vi "总磷氨氮MB_api.vi"(6 "Slave ID":u8=1, 7 "STEP":enum16{"open", "read", "write", "close"}(ring)=enum."read", 8 "Error in":errorcluster caption="Error in (no error)", 9 "values":u16[](array[numeric]), 10 "quantity":u16, 11 "starting address":u16 format="%04xH") -> (0 "error out":errorcluster, 2 "输出簇":T1, 3 "Registers":u16[](array[numeric]))   [LabVIEW 2016, in "氨氮.lvlib"]
uses:
  <vilib>/Plasmionique/MB Master/MB_ADU/MB_ADU.lvclass/MB_ADU.ctl
  <vilib>/Plasmionique/MB Master/MB_ADU/Read RX Data.vi
  <vilib>/Plasmionique/MB Master/MB_ADU/Read RX Timestamp.vi
  <vilib>/Plasmionique/MB Master/MB_ADU/Read Slave ID.vi
  <vilib>/Plasmionique/MB Master/MB_ADU/Read TX Data.vi
  <vilib>/Plasmionique/MB Master/MB_ADU/Read TX Timestamp.vi
  <vilib>/Plasmionique/MB Master/MB_Master_Serial/MB_Master_Serial.lvclass
  F:/Program Files/National Instruments/LabVIEW 2016/vi.lib/Plasmionique/MB Master/MB_Master/MB_Master.lvclass
  <vilib>/Plasmionique/MB Master/MB_ADU/MB_ADU.lvclass
  <vilib>/Plasmionique/MB Master/MB_Master/MB_Master.lvclass
  <vilib>/Plasmionique/MB Master/MB Master.lvlib
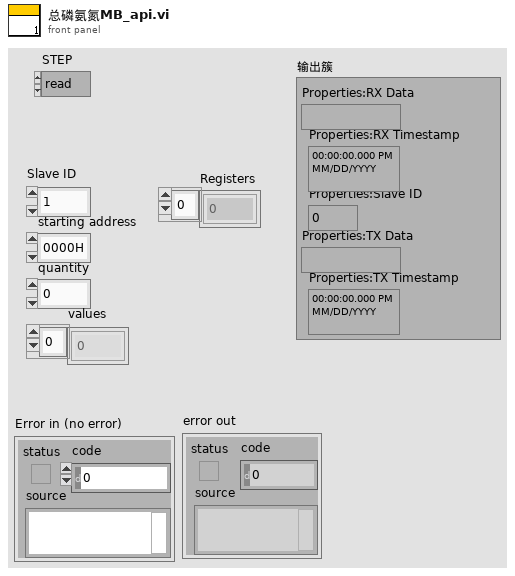
[diagram p1: front panel]
types:
  T1 = cluster{"Properties:RX Data":string, "Properties:RX Timestamp":timestamp, "Properties:Slave ID":u8, "Properties:TX Data":string, "Properties:TX Timestamp":timestamp}
  T2 = cluster{"baud rate (bps)":u32, "stop bits":u16, "parity":u16, "flow control":u16, "timeout":u32, "retries":i32}
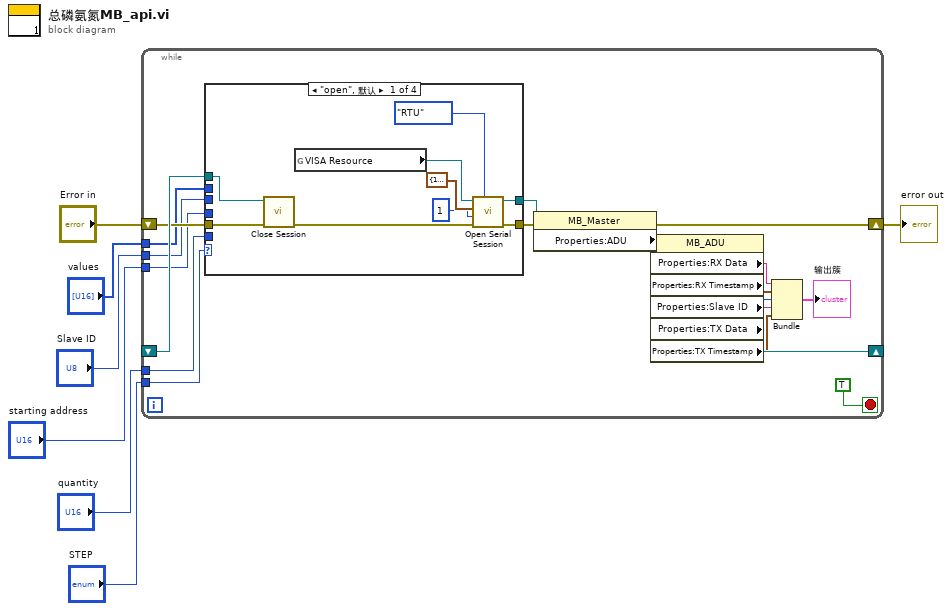
[diagram p0: block diagram]
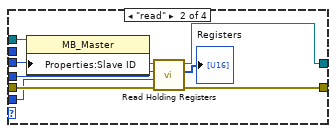
[diagram p2: hidden frame]
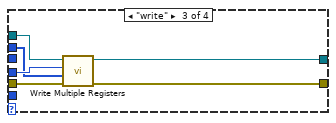
[diagram p3: hidden frame]
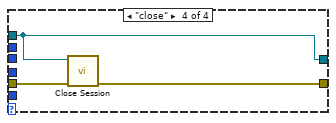
[diagram p4: hidden frame]
diagram:
  n1 = while {
    shift-right: [w19] -> _
    shift-left: _ -> [w26]
    shift-right: [w17] -> w6
    shift-left: "Error in" -> [w25]
    tunnel: "Slave ID" -> [w24]
    tunnel: "starting address" -> [w23]
    tunnel: "quantity" -> [w22]
    tunnel: "STEP" -> [w21]
    tunnel: "values" -> [w9]
    stop <- TRUE stop-if-true
    n2 = case shown="\"open\", 默认" w21 {
      tunnel: w26 -> [w30 w37 w48 w51]
      tunnel: w25 -> [w29 w44 w50 w53]
      tunnel: [w31 w43 w47 w51] -> w20
      tunnel: [w33 w42 w49 w52] -> w18
      tunnel: w24 -> [_ w40 _ _]
      tunnel: w23 -> [_ w39 w46 _]
      tunnel: w22 -> [_ w38 _ _]
      tunnel: w9 -> [_ _ w45 _]
      frame "open", Default {
        n3 = call-dynamic "Close Session.vi"("error in (no error)"=w29, "MB session in"=w30) -> ("error out"=w28:errorcluster)  [unwired: 9 in]
        n4 = global read "VAR总磷氨氮全局变量.vi" "VISA Resource"() -> (w27:refnum<visa-resource-name>)
        n5 = call <vilib>:"Open Serial Session.vi"("Mode (RTU)"=enum16{"RTU", "ASCII"}."RTU", "Error in"=w28, "Slave ID"=u8 1, "Serial Config"=T2 {"baud rate (bps)"=115200, "stop bits"=10, "parity"=0, "flow control"=0, "timeout"=100, "retries"=1}, "VISA Resource"=w27) -> ("Error out"=w33:errorcluster, "MB_Serial session"=w31:refnum<class "MB_Master_Serial.lvclass">)  [unwired: 5 in]
      }
      frame "read" {
        n6 = property class="MB_Master"(reference=w37, "Properties:Slave ID"=w40) -> (reference out=w36:refnum<class "MB_Master.lvclass">)  [unwired: 1 in, 1 out]
        n7 = call <vilib>:"Read Holding Registers.vi"("error in (no error)"=w44, "quantity"=w38, "starting address"=w39, "MB session in"=w36) -> ("error out"=w42:errorcluster, "Registers"=→"Registers":u16[], "MB session out"=w43:refnum<class "MB_Master.lvclass">)  [unwired: 5 in]
      }
      frame "write" {
        n8 = call <vilib>:"Write Multiple Registers.vi"("error in (no error)"=w50, "values"=w45, "starting address"=w46, "MB session in"=w48) -> ("error out"=w49:errorcluster, "MB session out"=w47:refnum<class "MB_Master.lvclass">)  [unwired: 6 in]
      }
      frame "close" {
        n9 = call-dynamic "Close Session.vi"("error in (no error)"=w53, "MB session in"=w51) -> ("error out"=w52:errorcluster)  [unwired: 9 in]
      }
    }
    n10 = property class="MB_Master"(reference=w20, error in=w18) -> (reference out=w19:refnum<class "MB_Master.lvclass">, error out=w17:errorcluster, "Properties:ADU"=w16:refnum<class "MB_ADU.lvclass">)
    n11 = property class="MB_ADU"(reference=w16) -> ("Properties:RX Data"=w15:string, "Properties:RX Timestamp"=w14:timestamp, "Properties:Slave ID"=w13:u8, "Properties:TX Data"=w12:string, "Properties:TX Timestamp"=w11:timestamp)  [unwired: 1 in, 2 out]
    n12 = Bundle("Properties:RX Data"=w15, "Properties:RX Timestamp"=w14, "Properties:Slave ID"=w13, "Properties:TX Data"=w12, "Properties:TX Timestamp"=w11) -> (→"输出簇":T1)  [unwired: 1 in]
  }
  "error out" <- w6
